vi "WSVCAP SHL Host TL I2C Read - Multiple Device.vi"(0 "Bytes to Read (1-4)":u8=4 min=1 max=4 step=1, 5 "Sub Address [U8]":u8=191 format="%.0x", 11 "error in":errorcluster, 13 "Log (T)":bool=TRUE) -> (4 "C1:1-16 Read Data [U8]":u8[][](array[numeric]) format="%.0x", 6 "C2:1-16 Read Data [U8]":u8[][](array[numeric]) format="%.0x", 8 "C3:1-16 Read Data [U8]":u8[][](array[numeric]) format="%.0x", 15 "error out":errorcluster)   [LabVIEW 2012]
panel:
  in  "DUT Mask Array (All)":bool[][](array[boolean])=[[TRUE, TRUE, TRUE, TRUE, TRUE, TRUE, TRUE, TRUE, TRUE, TRUE, TRUE, TRUE, TRUE, TRUE, TRUE, TRUE], [TRUE, TRUE, TRUE, TRUE, TRUE, TRUE, TRUE, TRUE, TRUE, TRUE, TRUE, TRUE, TRUE, TRUE, TRUE, TRUE], [TRUE, TRUE, TRUE, TRUE, TRUE, TRUE, TRUE, TRUE, TRUE, TRUE, TRUE, TRUE, TRUE, TRUE, TRUE, TRUE]]
  out "Socket Mask [U32]":u64=1 format="%08x"
  out "Data Headers":u8[](array[numeric])=[1, 2, 3, 4, 5, 6, 7, 8, 9, 10, 11, 12, 12, 14, 15, 16]
  # "DUT 01"
  # "DUT 02"
  # "DUT 03"
  # "DUT 04"
  # "DUT 05"
  # "DUT 06"
  # "DUT 07"
  # "DUT 08"
  # "DUT 09"
  # "DUT 10"
  # "DUT 11"
  # "DUT 12"
  # "DUT 13"
  # "DUT 14"
  # "DUT 15"
  # "DUT 16"
  # "C1"
  # "C2"
  # "C3"
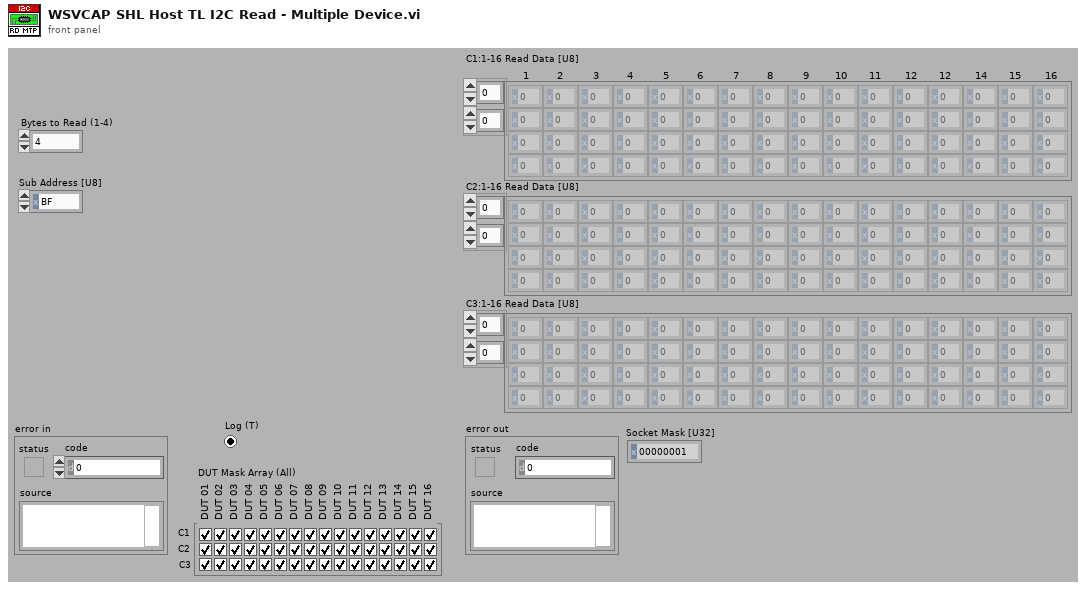
[diagram p1: front panel]
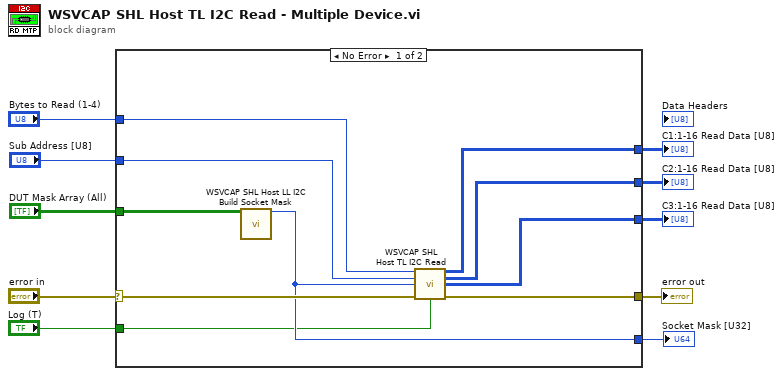
[diagram p0: block diagram]
diagram:
  n1 = case shown="No Error" "error in" {
    selector: "error in" -> [w19 w21]
    tunnel: [w20 w21] -> w10
    tunnel: "Bytes to Read (1-4)" -> [w18 _]
    tunnel: "Sub Address [U8]" -> [w17 _]
    tunnel: [w14 _] -> w6
    tunnel: [w16 _] -> w5
    tunnel: [w15 _] -> w4
    tunnel: "DUT Mask Array (All)" -> [w13 _]
    tunnel: "Log (T)" -> [w12 _]
    tunnel: [w11 _] -> w1
    frame No Error {
      n2 = call "WSVCAP SHL Host LL I2C Build Socket Mask.vi"("DUT Mask Array"=w13) -> ("Socket Mask [U64]"=w14:u64)  [unwired: 13 in, 1 out]
      n3 = call "WSVCAP SHL Host TL I2C Read.vi"("Bytes to Read"=w18, "Sub Address [U8]"=w17, "Socket Mask [U64]"=w14, "error in"=w19, "Log (T)"=w12) -> ("C1 Read Data Out"=w16:u8[][], "C2 Read Data Out"=w15:u8[][], "C3 Read Data Out"=w11:u8[][], "error out"=w20:errorcluster)  [unwired: 7 in]
    }
    frame Error {
    }
  }
  "error out" <- w10
  "Socket Mask [U32]" <- w6
  "C1:1-16 Read Data [U8]" <- w5
  "C2:1-16 Read Data [U8]" <- w4
  "C3:1-16 Read Data [U8]" <- w1
